vi "SW_Get_save_paths.vi"(3 "error in (no error)":errorcluster, 4 "Input cluster of paths":T1, 5 "Final file name prefix":string="Track", 6 "Temporary file name prefix":string="TrackTemp") -> (0 "error out":errorcluster, 1 "Saved track name":string, 2 "Output cluster of paths":T2)   [LabVIEW 2018, in "Tracker.lvlib"]
uses:
  <vilib>/Utility/sysdir.llb/System Directory Type.ctl
  Tracker.lvlib
panel:
  out "TDMS output path":path
  out "Final output path":path
  out "Layout picture output path":path
  out "Recording settings output path":path
  out "Density map array output path":path
  out "date/time string":string
  out "Temporary file output path":path
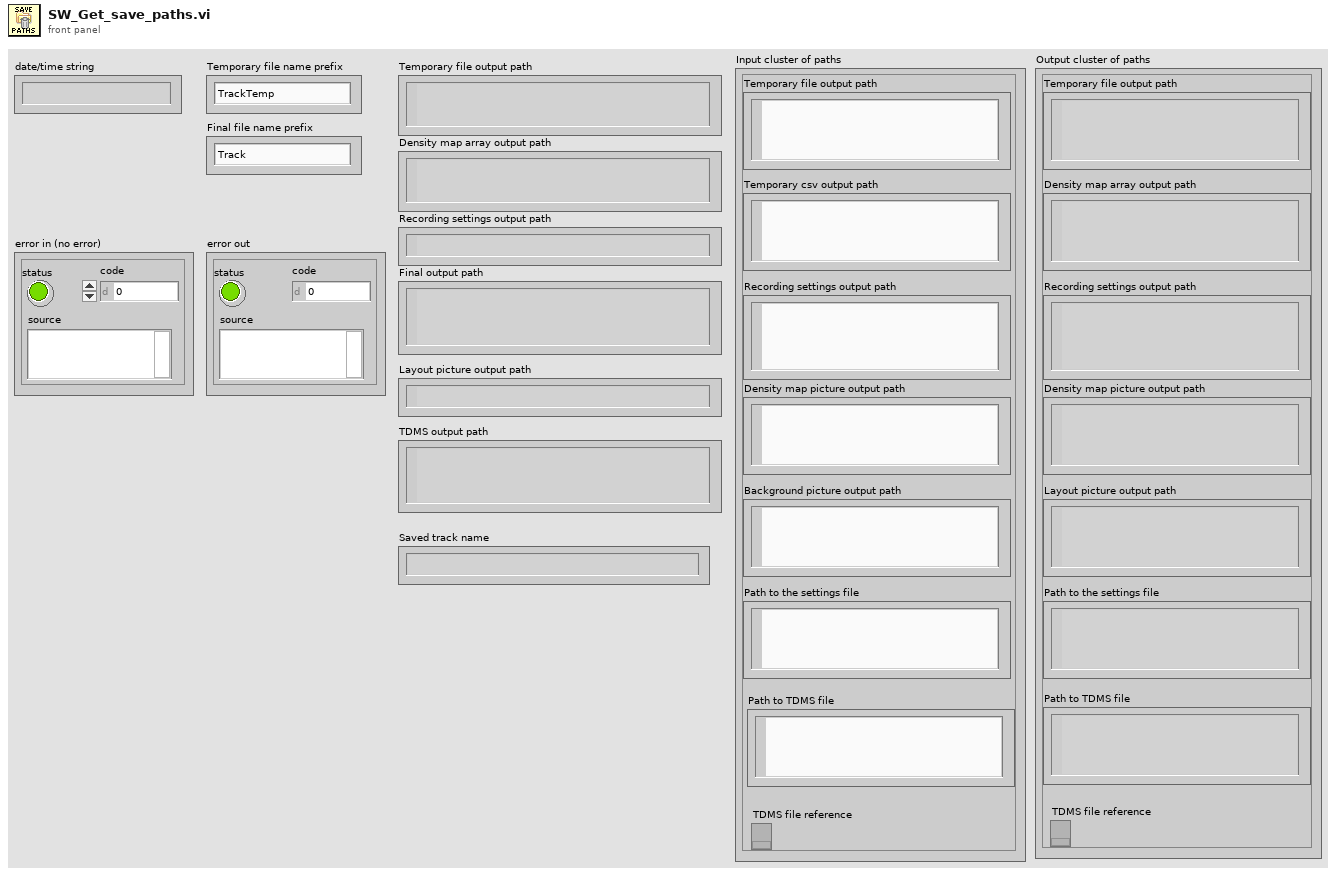
[diagram p1: front panel]
types:
  T1 = cluster{"Temporary file output path":path, "Temporary csv output path":path, "Recording settings output path":path, "Density map picture output path":path, "Background picture output path":path, "Path to the settings file":path, "Path to TDMS file":path, "TDMS file reference":refnum<k34>}
  T2 = cluster{"Temporary file output path":path, "Density map array output path":path, "Recording settings output path":path, "Density map picture output path":path, "Layout picture output path":path, "Path to the settings file":path, "Path to TDMS file":path, "TDMS file reference":refnum<k34>}
  T3 = enum16{"big-endian, network order", "native, host order", "little-endian"}
  T4 = enum16{"open", "open or create", "create or replace", "create", "open (read-only)"}
  T5 = typedef "System Directory Type.ctl" = i32
  T6 = cluster{path, path, path, path, path, "Path to the settings file":path, path, "tdms file out":refnum<k34>}
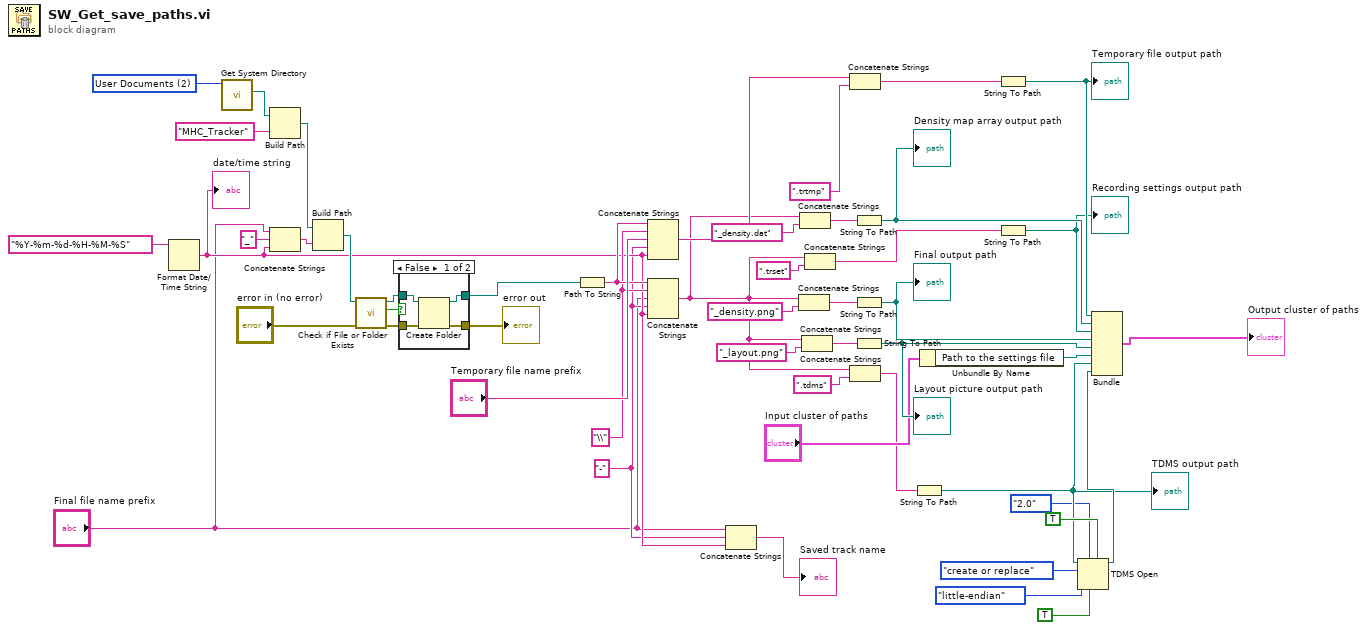
[diagram p0: block diagram]
diagram:
  w48 = T5 2 items=["User Home"=0, "User Desktop"=1, "User Documents"=2, "User Application Data"=3, "User Preferences"=4, "User Temporary"=5, "Public Documents"=6, "Public Application Data"=7, "Public Preferences"=8, "Public Cache"=13, "System Core Libraries"=9, "System Installed Libraries"=10, "Application Files"=11, "Boot Volume Root"=12] ("system directory type")
  w6 = "-" ("string")
  w35 = "\\" ("string")
  n1 = Format Date/Time String(time format string (%c)="%Y-%m-%d-%H-%M-%S") -> (date/time string=w7:string)  [unwired: 2 in]
  "date/time string" <- w7
  n2 = call <vilib>:"Get System Directory.vi"("system directory type"=w48) -> ("system directory"=w46:path)  [unwired: 10 in]
  n3 = Build Path(base path=w46, name or relative path="MHC_Tracker" ("string")) -> (appended path=w23:path)
  n4 = Concatenate Strings("Final file name prefix", "_" ("string"), w7) -> (w20:string)
  n5 = Build Path(base path=w23, name or relative path=w20) -> (appended path=w22:path)
  n6 = call <vilib>:"Check if File or Folder Exists.vi"("error in (no error)"="error in (no error)", "path"=w22) -> ("error out"=w43:errorcluster, "file or folder exists?"=w45:bool, "dup path"=w44:path)  [unwired: 7 in]
  n7 = case shown="False" w45 {
    tunnel: w44 -> [w53 w56]
    tunnel: w43 -> [w54 w55]
    tunnel: [w51 w56] -> w25
    tunnel: [w52 w55] -> w24
    frame False {
      n8 = Create Folder(path (use dialog)=w53, error in=w54) -> (created path=w51:path, error out=w52:errorcluster)  [unwired: 1 in, 1 out]
    }
    frame True {
    }
  }
  "error out" <- w24
  n9 = Path To String(path=w25) -> (string=w36:string)
  n10 = Concatenate Strings(w36, w35, "Temporary file name prefix", w6, w7) -> (w28:string)
  n11 = Concatenate Strings(w36, w35, "Final file name prefix", w6, w7) -> (w1:string)
  n12 = Concatenate Strings("Final file name prefix", w6, w7) -> (→"Saved track name":string)
  n13 = Concatenate Strings(w1, "_density.png" ("string")) -> (w38:string)
  n14 = Concatenate Strings(w1, "_density.dat" ("string")) -> (w39:string)
  n15 = Concatenate Strings(w1, "_layout.png" ("string")) -> (w29:string)
  n16 = Concatenate Strings(w1, ".trset" ("string")) -> (w27:string)
  n17 = Concatenate Strings(w28, ".trtmp" ("string")) -> (w41:string)
  n18 = Concatenate Strings(w1, ".tdms" ("string")) -> (w14:string)
  n19 = String To Path(string=w39) -> (path=w33:path)
  "Density map array output path" <- w33
  n20 = String To Path(string=w38) -> (path=w31:path)
  "Final output path" <- w31
  n21 = String To Path(string=w29) -> (path=w30:path)
  "Layout picture output path" <- w30
  n22 = String To Path(string=w14) -> (path=w9:path)
  "TDMS output path" <- w9
  n23 = Unbundle By Name("Input cluster of paths") -> ("Path to the settings file"=w17:path)
  n24 = String To Path(string=w41) -> (path=w34:path)
  "Temporary file output path" <- w34
  n25 = String To Path(string=w27) -> (path=w32:path)
  "Recording settings output path" <- w32
  n26 = TDMS Open(5:TRUE ("create index file? (T)"), 6:TRUE ("disable buffering? (T)"), 7:enum16{"1.0", "2.0"}."2.0" ("file format version (2.0)"), 9:T3."little-endian" ("byte order (2:little-endian)"), 10:T4."create or replace" ("operation (0:open)"), 11:w9) -> (3:w10:refnum<k34>)  [unwired: 1 in, 1 out]
  n27 = Bundle(w34, w33, w32, w31, w30, "Path to the settings file"=w17, w9, "tdms file out"=w10) -> (→"Output cluster of paths":T6)  [unwired: 1 in]
